vi "Memory.Truncate I32.vi"(11 "I32":i32) -> (3 "truncated I32":i32)   [LabVIEW 2016, in "LabVIEW Memory Manager.lvlib"]
uses:
  LabVIEW Memory Manager.lvlib
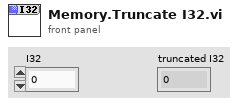
[diagram p1: front panel]
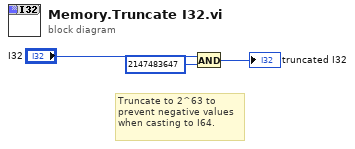
[diagram p0: block diagram]
diagram:
  # "Truncate to 2^63 to prevent negative values when casting to I64."
  n1 = And(x="I32", y=2147483647) -> (x .and. y?=→"truncated I32":i32)
